vi "Look for Optical Measurement.vi"(2 "Instrument Steps in":T2) -> (0 "Optical Measurement?":bool, 1 "Enabled":T1(ring))   [LabVIEW 2014]
uses:
  Instrument Sequence/Instrument Steps.ctl
  Instrument Sequence/Action.ctl
  Instrument Sequence/Instrument List.ctl
panel:
  # "LICENSED MATERIALS – PROPERTY OF IBM\nCopyright IBM Corp. 2016,\nALL RIGHTS RESERVED"
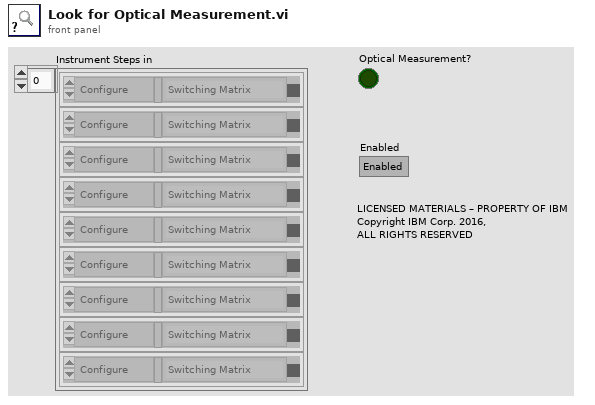
[diagram p1: front panel]
types:
  T1 = enum8{"Enabled", "Disabled", "Disabled and Grayed Out"}
  T2 = typedef "Instrument Steps.ctl" = cluster{"Action":T3, "Configuration":variant, "Instrument":T4, "Status":enum8{"False", "True", "Mixed"}}[]
  T3 = typedef "Action.ctl" = enum32{"Configure", "Measure"}
  T4 = typedef "Instrument List.ctl" = enum32{"Unknown Instrument", "Switching Matrix", "Parameter Analyzer", "Optical Spectrometer", "Optoelectronic", "Autofocus"}
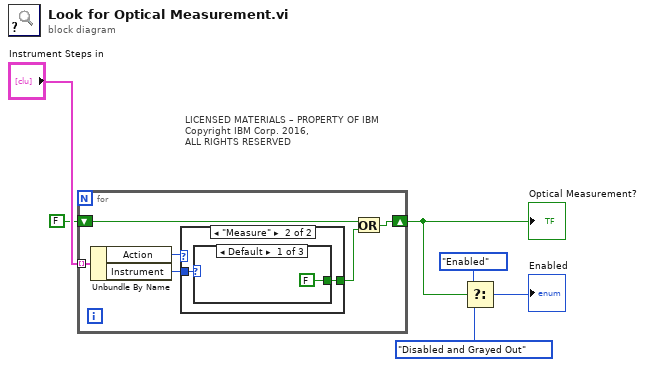
[diagram p0: block diagram]
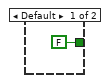
[diagram p2: hidden frame]
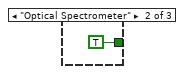
[diagram p3: hidden frame]
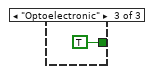
[diagram p4: hidden frame]
diagram:
  # "LICENSED MATERIALS – PROPERTY OF IBM\nCopyright IBM Corp. 2016,\nALL RIGHTS RESERVED"
  n1 = for {
    tunnel: "Instrument Steps in" -> [w10] mode=indexing
    shift-right: [w11] -> w4
    shift-left: FALSE -> [w12]
    n2 = Unbundle By Name(w10) -> ("Action"=w9:T3, "Instrument"=w8:T4)
    n3 = case shown="\"Measure\"" w9 {
      tunnel: w8 -> [_ w15]
      tunnel: [FALSE w14] -> w7
      frame Default {
      }
      frame "Measure" {
        n4 = case shown="Default" w15 {
          tunnel: [FALSE TRUE TRUE] -> w14
          frame Default {
          }
          frame "Optical Spectrometer" {
          }
          frame "Optoelectronic" {
          }
        }
      }
    }
    n5 = Or(x=w12, y=w7) -> (x .or. y?=w11:bool)
  }
  "Optical Measurement?" <- w4
  n6 = Select(t=T1."Enabled" ("Enabled 2"), s=w4, f=T1."Disabled and Grayed Out" ("Enabled 2")) -> (s? t:f=→"Enabled":T1)
